vi "正解.vi"(1 "Vc":dbl, 2 "Va":dbl, 3 "H":dbl, 4 "S0":dbl) -> (0 "投彈時間(k)":dbl)   [LabVIEW 2014]
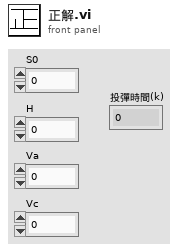
[diagram p1: front panel]
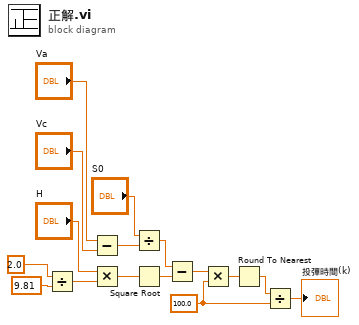
[diagram p0: block diagram]
diagram:
  w2 = 100.0 ("y")
  n1 = Divide(x=2.0, y=9.81) -> (x/y=w9:dbl)
  n2 = Subtract(x="Va", y="Vc") -> (x-y=w13:dbl)
  n3 = Multiply(x="H", y=w9) -> (x*y=w8:dbl)
  n4 = Divide(x="S0", y=w13) -> (x/y=w7:dbl)
  n5 = Square Root(x=w8) -> (sqrt(x)=w6:dbl)
  n6 = Subtract(x=w7, y=w6) -> (x-y=w5:dbl)
  n7 = Multiply(x=w5, y=w2) -> (x*y=w4:dbl)
  n8 = Round To Nearest(number=w4) -> (nearest integer value=w3:dbl)
  n9 = Divide(x=w3, y=w2) -> (x/y=→"投彈時間(k)":dbl)
